vi "set operation mode.vi"(8 "error in (no error)":errorcluster, 10 "Operating Mode (0: Int Synch, Continuously Running w SW Capture-Start)":T1 items=["Int Synch, Continuously Running w SW Capture-Start", "Int Synch, Continuously Running w HW Capture-Start", "Int Synch, Continuously Running w HW Capture-Enable", "Single Shot, Clean&Ready w ext. HW Trigger", "Ext Synch, Continuously Runnung w SW Capture-Start"], 11 "LineCCD in":refnum<class "LineCCD.lvclass">) -> (0 "error out":errorcluster, 3 "LineCCD out":refnum<class "LineCCD.lvclass">)   [LabVIEW 2012, in "LineCCD.lvclass"]
uses:
  LineCCD.lvclass
  <instrlib>/ALPHALAS CCD S Series/Public/Typedefs/Operating Mode.ctl
  LineCCD.lvclass/LineCCD.ctl
  <instrlib>/ALPHALAS CCD S Series/ALPHALAS CCD S Series.lvlib
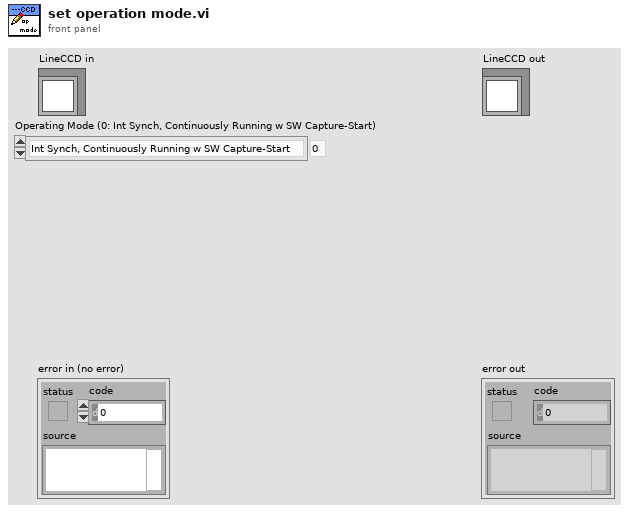
[diagram p1: front panel]
types:
  T1 = typedef "ALPHALAS CCD S Series.lvlib/Operating Mode.ctl" = u16
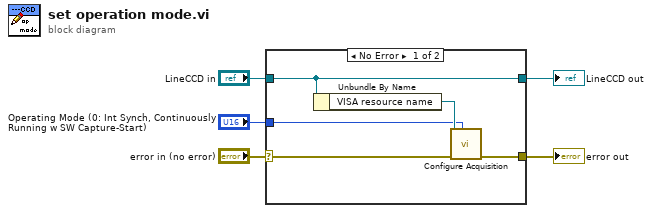
[diagram p0: block diagram]
diagram:
  n1 = case shown="No Error" "error in (no error)" {
    selector: "error in (no error)" -> [w8 w12]
    tunnel: [w7 w12] -> w4
    tunnel: [w9 w11] -> w2
    tunnel: "LineCCD in" -> [w9 w11]
    tunnel: "Operating Mode (0: Int Synch, Continuously Running w SW Capture-Start)" -> [w6 _]
    frame No Error {
      n2 = Unbundle By Name(w9) -> ("VISA resource name"=w10:refnum<visa-resource-name>)
      n3 = call <instrlib>:"Configure Acquisition.vi"("Operating Mode (0: Int Synch, Continuously Running w SW Capture-Start)"=w6, "error in (no error)"=w8, "VISA resource name"=w10) -> ("error out"=w7:errorcluster)  [unwired: 7 in, 1 out]
    }
    frame Error {
    }
  }
  "error out" <- w4
  "LineCCD out" <- w2
